vi "Ball at goalkeeper area.vi"(9 "Field defense":dbl[](array[numeric]), 10 "IA State":T1) -> (2 "Ball at goalkeeper area ?":bool)   [LabVIEW 2016]
uses:
  Core/AI Input.ctl
  Core/AI Robot.ctl
  Intel/Functions Enum.ctl
  Core/AI Ball.ctl
  Core/Field Size.ctl
  Core/AI Judge.ctl
  Intel/Command Enum.ctl
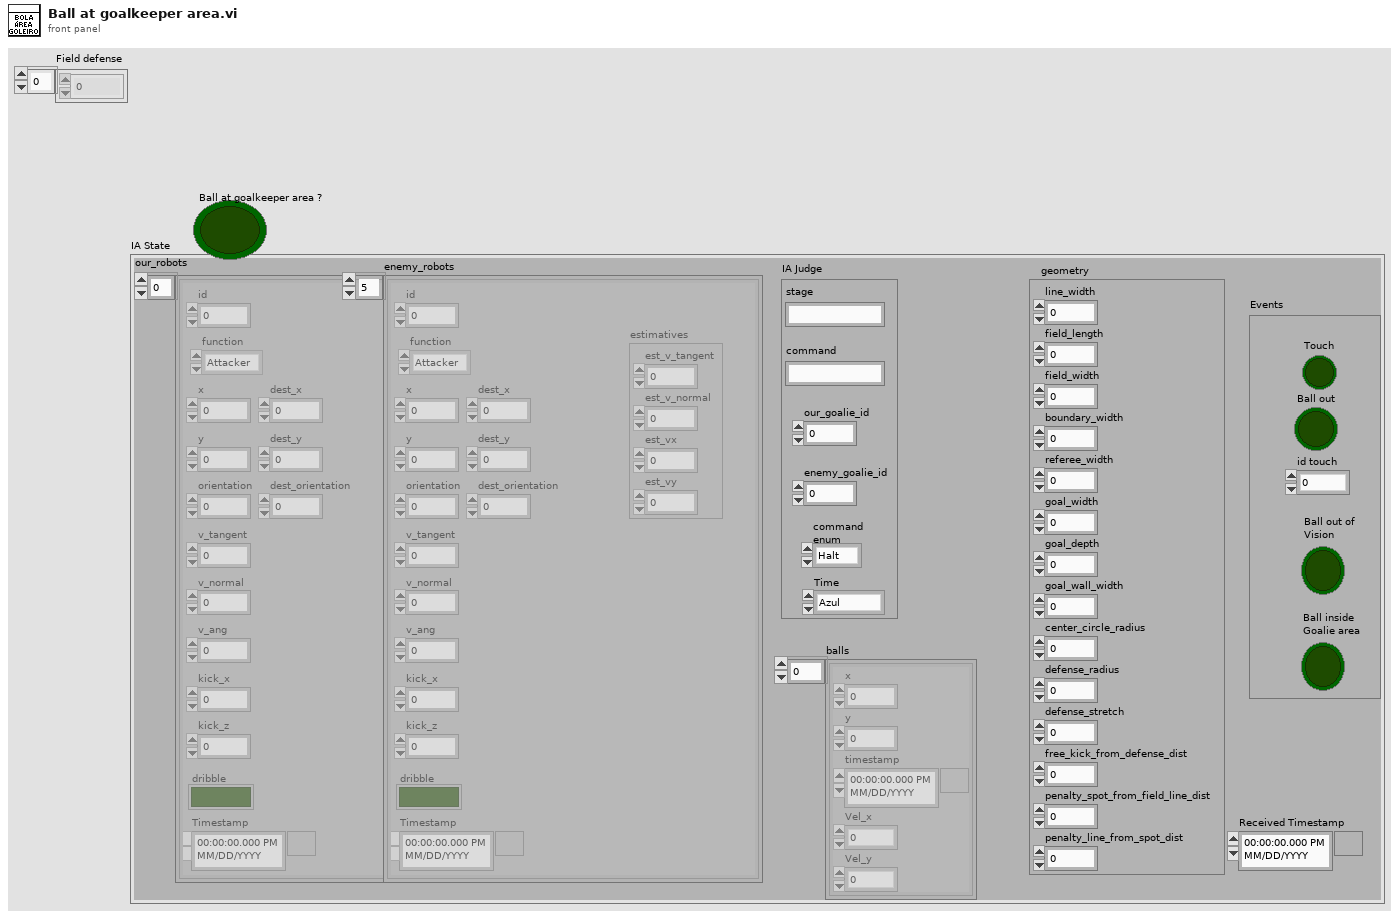
[diagram p1: front panel]
types:
  T1 = typedef "AI Input.ctl" = cluster{"our_robots":T2[], "enemy_robots":T2[], "balls":T4[], "geometry":T5, "IA Judge":T6, "Received Timestamp":timestamp, "Events":cluster{"Touch":bool, "Ball out":bool, "id touch":dbl, "Ball out of \nVision":bool, "Ball inside \nGoalie area":bool}}
  T2 = typedef "AI Robot.ctl" = cluster{"id":u32, "function":T3, "x":dbl, "y":dbl, "orientation":dbl, "v_tangent":dbl, "v_normal":dbl, "v_ang":dbl, "kick_x":dbl, "kick_z":dbl, "dribble":bool, "Timestamp":timestamp, "dest_x":dbl, "dest_y":dbl, "dest_orientation":dbl, "estimatives":cluster{"est_v_tangent":dbl, "est_v_normal":dbl, "est_vx":dbl, "est_vy":dbl}}
  T3 = typedef "Functions Enum.ctl" = enum16{"Attacker", "Goalie", "Defender", "Striker", "Goto 0", "Dummy", "ZigZag"}
  T4 = typedef "AI Ball.ctl" = cluster{"x":dbl, "y":dbl, "timestamp":timestamp, "Vel_x":dbl, "Vel_y":dbl}
  T5 = typedef "Field Size.ctl" = cluster{"line_width":u32, "field_length":u32, "field_width":u32, "boundary_width":u32, "referee_width":u32, "goal_width":u32, "goal_depth":u32, "goal_wall_width":u32, "center_circle_radius":u32, "defense_radius":u32, "defense_stretch":u32, "free_kick_from_defense_dist":u32, "penalty_spot_from_field_line_dist":u32, "penalty_line_from_spot_dist":u32}
  T6 = typedef "AI Judge.ctl" = cluster{"stage":string, "command":string, "our_goalie_id":dbl, "enemy_goalie_id":dbl, "command\nenum":T7, "Time":enum16{"Azul", "Amarelo"}}
  T7 = typedef "Command Enum.ctl" = enum16{"Halt", "Stop", "Force Start", "PKA Normal Start", "Prepare Kickoff Ally", "PKE Normal Start", "Prepare Kickoff Enemy", "Prepare Penalty Ally", "PPA Normal Start", "Prepare Penalty Enemy", "PPE Normal Start", "Direct Free Enemy", "Direct Free Ally", "Indirect Free Enemy", "Indirect Free Ally", "Timeout Enemy", "Timeout Ally", "Goal Enemy", "Goal Ally", "Ball Placement Enemy", "Ball Placement Ally", "None"}
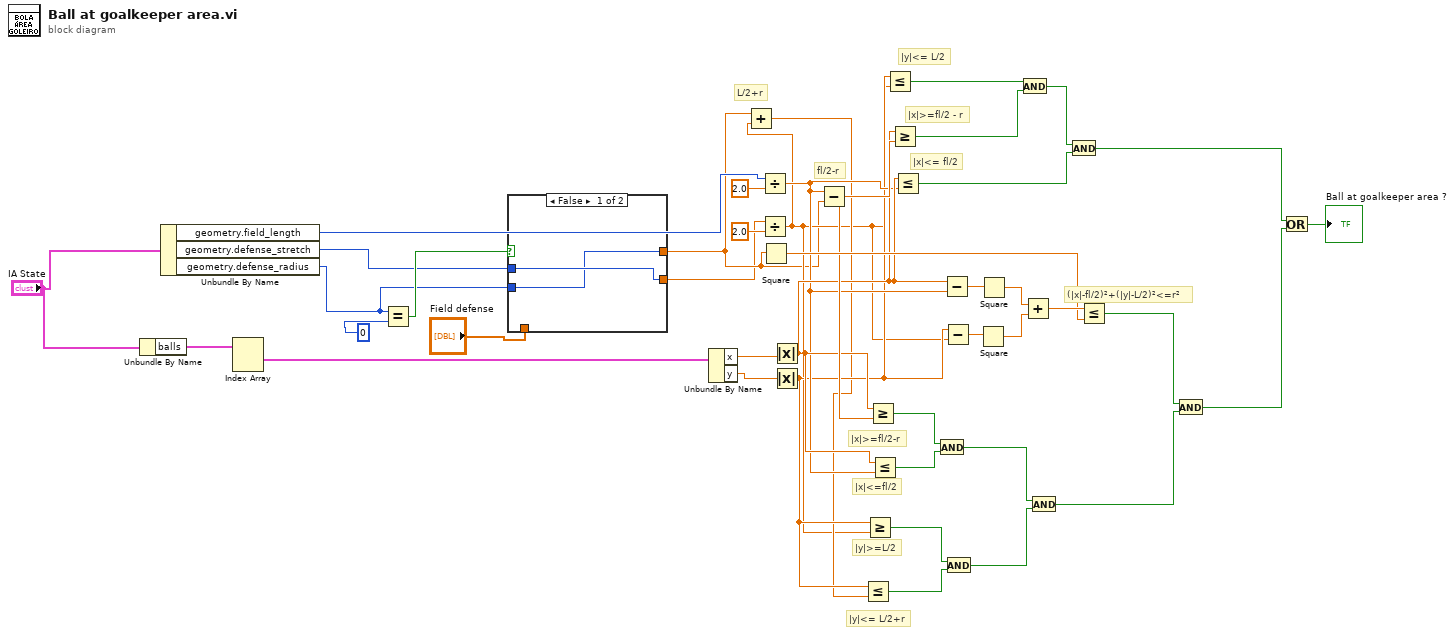
[diagram p0: block diagram]
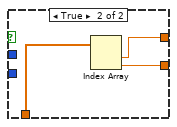
[diagram p2: hidden frame]
diagram:
  # "|y|<= L/2+r"
  # "L/2+r"
  # "|y|>=L/2"
  # "|x|<=fl/2"
  # "|x|>=fl/2-r"
  # "fl/2-r"
  # "(|x|-fl/2)²+(|y|-L/2)²<=r²"
  # "|x|<= fl/2"
  # "|x|>=fl/2 - r"
  # "|y|<= L/2"
  n1 = Unbundle By Name("IA State") -> ("balls"=w42:T4[])
  n2 = Unbundle By Name("IA State") -> ("geometry.field_length"=w35:u32, "geometry.defense_stretch"=w2:u32, "geometry.defense_radius"=w1:u32)
  n3 = Index Array(array=w42) -> (element #1=w41:T4)  [unwired: 2 in, 1 out]
  n4 = Equal?(x=w1, y=u32 0) -> (x = y?=w5:bool)
  n5 = case shown="False" w5 {
    tunnel: [w43 w47] -> w4
    tunnel: [w44 w46] -> w3
    tunnel: "Field defense" -> [_ w45]
    tunnel: w2 -> [w44 _]
    tunnel: w1 -> [w43 _]
    frame False {
    }
    frame True {
      n6 = Index Array(array=w45) -> (element #1=w47:dbl, element #2=w46:dbl)  [unwired: 2 in]
    }
  }
  n7 = Unbundle By Name(w41) -> ("x"=w38:dbl, "y"=w39:dbl)
  n8 = Divide(x=w35, y=2.0) -> (x/y=w20:dbl)
  n9 = Divide(x=w3, y=2.0) -> (x/y=w8:dbl)
  n10 = Add(x=w4, y=w8) -> (x+y=w18:dbl)
  n11 = Square(x=w4) -> (x^2=w25:dbl)
  n12 = Absolute Value(x=w38) -> (abs(x)=w23:dbl)
  n13 = Absolute Value(x=w39) -> (abs(x)=w19:dbl)
  n14 = Subtract(x=w20, y=w4) -> (x-y=w24:dbl)
  n15 = Less Or Equal?(x=w19, y=w18) -> (x <= y?=w16:bool)
  n16 = Greater Or Equal?(x=w19, y=w8) -> (x >= y?=w17:bool)
  n17 = Greater Or Equal?(x=w23, y=w24) -> (x >= y?=w22:bool)
  n18 = Less Or Equal?(x=w23, y=w20) -> (x <= y?=w21:bool)
  n19 = Less Or Equal?(x=w19, y=w8) -> (x <= y?=w34:bool)
  n20 = Greater Or Equal?(x=w23, y=w24) -> (x >= y?=w33:bool)
  n21 = Less Or Equal?(x=w23, y=w20) -> (x <= y?=w31:bool)
  n22 = And(x=w22, y=w21) -> (x .and. y?=w15:bool)
  n23 = Subtract(x=w23, y=w20) -> (x-y=w30:dbl)
  n24 = Subtract(x=w19, y=w8) -> (x-y=w29:dbl)
  n25 = And(x=w17, y=w16) -> (x .and. y?=w14:bool)
  n26 = Square(x=w29) -> (x^2=w27:dbl)
  n27 = Square(x=w30) -> (x^2=w28:dbl)
  n28 = And(x=w34, y=w33) -> (x .and. y?=w32:bool)
  n29 = Add(x=w28, y=w27) -> (x+y=w26:dbl)
  n30 = And(x=w15, y=w14) -> (x .and. y?=w12:bool)
  n31 = And(x=w32, y=w31) -> (x .and. y?=w11:bool)
  n32 = Less Or Equal?(x=w26, y=w25) -> (x <= y?=w13:bool)
  n33 = And(x=w13, y=w12) -> (x .and. y?=w10:bool)
  n34 = Or(x=w11, y=w10) -> (x .or. y?=→"Ball at goalkeeper area ?":bool)
